vi "RefnameToString.vi"(1 "Enum":T1) -> (0 "Refname":string)   [LabVIEW 2013]
uses:
  RefnameEnum.ctl
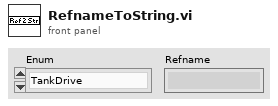
[diagram p1: front panel]
types:
  T1 = typedef "RefnameEnum.ctl" = enum16{"TankDrive", "Controller1", "Controller2"}
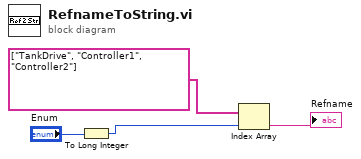
[diagram p0: block diagram]
diagram:
  n1 = To Long Integer(number="Enum") -> (32bit integer=w2:i32)
  n2 = Index Array(array=string[] ["TankDrive", "Controller1", "Controller2"], index=w2) -> (element=→"Refname":string)
